vi "Get Temperature Corrected Permeation Rate.vi"(8 "error in":errorcluster, 11 "Owlstone GEN-SYS in":refnum<class "Owlstone GEN-SYS.lvclass">) -> (0 "error out":errorcluster, 2 "Permeation Rate":dbl, 3 "Owlstone GEN-SYS out":refnum<class "Owlstone GEN-SYS.lvclass">)   [LabVIEW 2011, in "Owlstone GEN-SYS.lvclass"]
uses:
  Owlstone GEN-SYS.lvclass
  Owlstone GEN-SYS.lvclass/Owlstone GEN-SYS.ctl
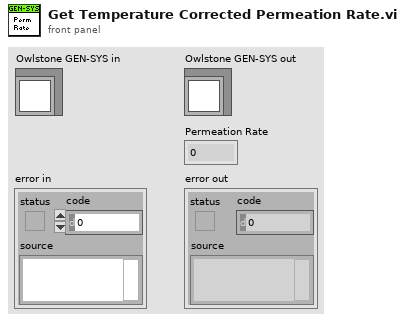
[diagram p1: front panel]
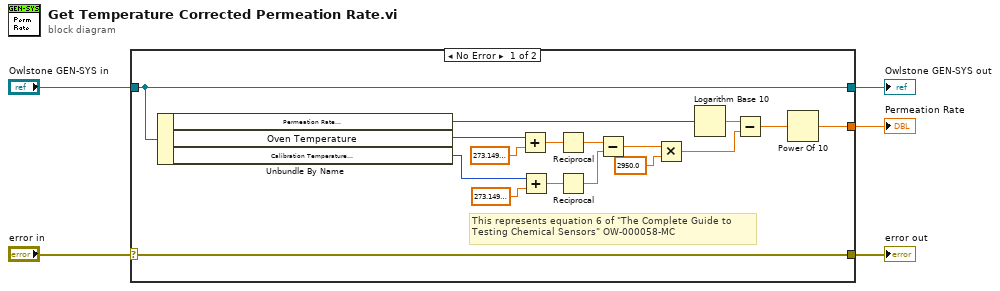
[diagram p0: block diagram]
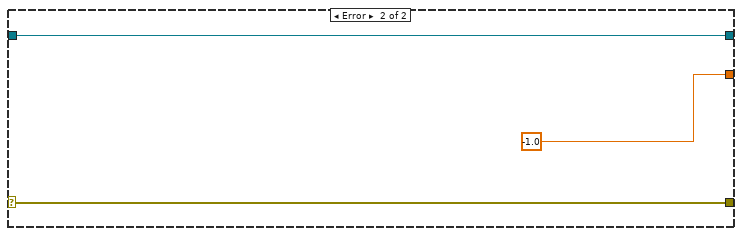
[diagram p2: hidden frame]
diagram:
  n1 = case shown="No Error" "error in" {
    selector: "error in" -> [w22 w25]
    tunnel: [w22 w25] -> w4
    tunnel: [w21 w24] -> w2
    tunnel: "Owlstone GEN-SYS in" -> [w21 w24]
    tunnel: [w6 -1.0] -> w1
    frame No Error {
      # "This represents equation 6 of \"The Complete Guide to\nTesting Chemical Sensors\" OW-000058-MC"
      n2 = Unbundle By Name(w21) -> ("Permeation Rate \n(ng/min)"=w10:i32, "Oven Temperature"=w16:i32, "Calibration Temperature\n(Celcius)"=w14:i32)
      n3 = Add(x=w16, y=sgl 273.15) -> (x+y=w12:sgl)
      n4 = Add(x=w14, y=sgl 273.15) -> (x+y=w11:sgl)
      n5 = Reciprocal(x=w12) -> (1/x=w20:sgl)
      n6 = Reciprocal(x=w11) -> (1/x=w19:sgl)
      n7 = Subtract(x=w20, y=w19) -> (x-y=w18:sgl)
      n8 = Multiply(x=w18, y=2950.0) -> (x*y=w8:dbl)
      n9 = Logarithm Base 10(1:w10) -> (0:w9:dbl)
      n10 = Subtract(x=w9, y=w8) -> (x-y=w7:dbl)
      n11 = Power Of 10(x=w7) -> (10^x=w6:dbl)
    }
    frame Error {
    }
  }
  "error out" <- w4
  "Owlstone GEN-SYS out" <- w2
  "Permeation Rate" <- w1
